vi "Sub Initialize.vi"(8 "error in (no error)":errorcluster, 11 "RP I-V in":refnum<class "RP I-V.lvclass">) -> (0 "error out":errorcluster, 2 "Initialize Result":refnum<class "Acquired Result.lvclass">, 3 "RP I-V out":refnum<class "RP I-V.lvclass">)   [LabVIEW 2016, in "RP I-V.lvclass"]
uses:
  RP I-V.lvclass
  C:/github/Measure_core/Pulse Recorders/Pulse Recorder/Pulse Recorder.lvclass
  Measure_core/Results/Acquired Result/Acquired Result.lvclass
  NHMFL_Core/Libraries/Red Pitaya/RP Core/Rep Pitaya I-V driver/RP I-V Driver.lvclass
  C:/github/NHMFL_Core/Libraries/Instruments/Pulse Driver/Pulse Driver.lvclass
  Measure_core/Pulse Recorders/Pulse Recorder/Read Pulse driver.vi
  Measure_core/Pulse Recorders/Pulse Recorder/Write Pulse driver.vi
  NHMFL_Core/Libraries/Instruments/Pulse Driver/Pulse Driver.lvclass
  Measure_core/Pulse Recorders/Pulse Recorder/Pulse Recorder.lvclass
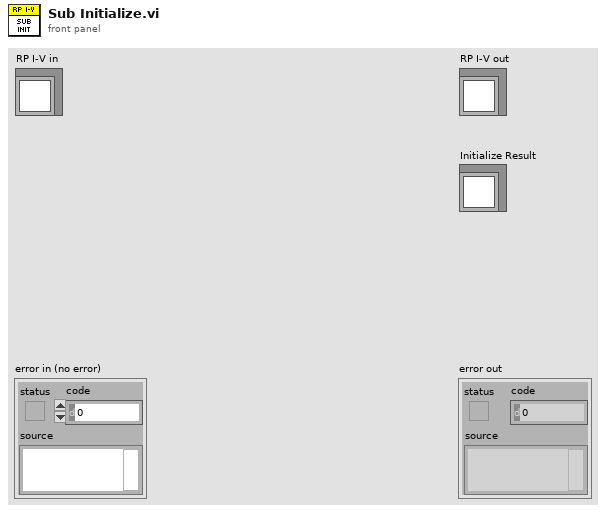
[diagram p1: front panel]
types:
  T1 = typedef "RP I-V Configuration.ctl" = cluster{"Recorder":T2, "I-V parameters":T3}
  T2 = typedef "Pusle Driver Configuration.ctl" = cluster{"Pre-trigger duration":dbl, "Post-trigger duration":dbl, "Rate":dbl, "Ranges":dbl[], "Re-name channels":string[], "Active channels":string, "External clock":bool}
  T3 = typedef "I-V parameters.ctl" = cluster{"Start magnitude":dbl, "Magnitude increment":dbl, "Number of pulses":i32, "Baseline length":i32, "Ramp length":i32, "Top  length":i32, "Threshold ":dbl, "Processing Delay":u16, "Valhalla range":dbl, "Interpolation":i32}
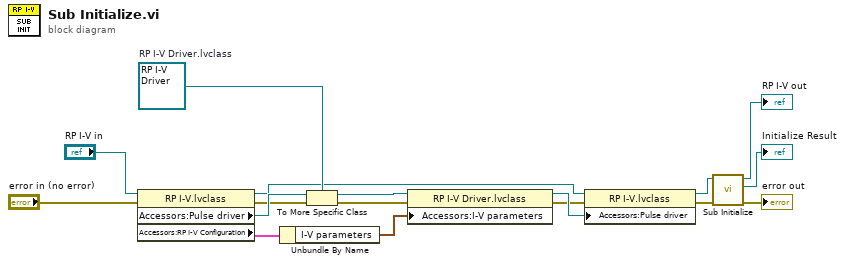
[diagram p0: block diagram]
diagram:
  w11 = refnum<class "RP I-V Driver.lvclass"> refnum  # RP I-V Driver.lvclass
  n1 = property class="RP I-V.lvclass"(reference="RP I-V in", error in="error in (no error)") -> (reference out=w1:refnum<class "RP I-V.lvclass">, error out=w8:errorcluster, "Accessors:Pulse driver"=w12:refnum<class "Pulse Driver.lvclass">, "Accessors:RP I-V Configuration"=w7:T1)
  n2 = Unbundle By Name(w7) -> ("I-V parameters"=w6:T3)
  n3 = To More Specific Class(target class=w11, reference=w12, error in=w8) -> (specific class reference=w10:refnum<class "RP I-V Driver.lvclass">, error out=w9:errorcluster)
  n4 = property class="RP I-V Driver.lvclass"(reference=w10, error in=w9, "Accessors:I-V parameters"=w6) -> (reference out=w5:refnum<class "RP I-V Driver.lvclass">, error out=w4:errorcluster)
  n5 = property class="RP I-V.lvclass"(reference=w1, error in=w4, "Accessors:Pulse driver"=w5) -> (reference out=w3:refnum<class "RP I-V.lvclass">, error out=w2:errorcluster)
  n6 = call-parent "Sub Initialize.vi"("error in (no error)"=w2, "Instrument Recorder in"=w3) -> ("error out"=→"error out":errorcluster, "Initialize Result"=→"Initialize Result":refnum<class "Acquired Result.lvclass">, "Instrument Recorder out"=→"RP I-V out":refnum<class "RP I-V.lvclass">)  [unwired: 7 in]
